vi "Get Temp Power Stage.vi"(8 "error in":errorcluster, 10 "?":T1, 11 "HSU MCU V2 Monitor CFG in":refnum<class "HSU MCU V2 CFG.lvclass">) -> (0 "error out":errorcluster, 2 "Temperature":dbl format="%#_g °C", 3 "HSU MCU V2 Monitor CFG out":refnum<class "HSU MCU V2 CFG.lvclass">)   [LabVIEW 2024, in "HSU MCU V2 CFG.lvclass"]
doc: "PCB temperature of MCUs power stage/MOSFETS"
uses:
  HSU MCU V2 CFG.lvclass
  MCU Selector.ctl
  HSU MCU V2 CFG.lvclass/HSU MCU V2 CFG.ctl
  Protocols/ICAN/ICAN.lvclass
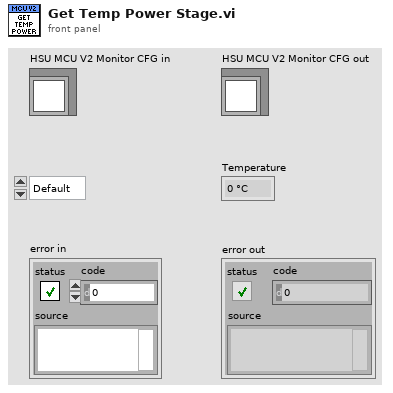
[diagram p1: front panel]
types:
  T1 = typedef "MCU Selector.ctl" = enum16{"Default", "MCU1", "MCU2", "MCU3", "MCU4", "MCU5", "MCU6", "MCU7", "MCU8", "ALL"}
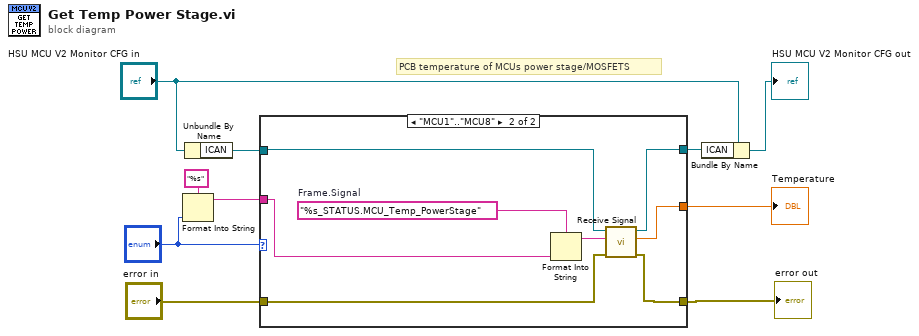
[diagram p0: block diagram]
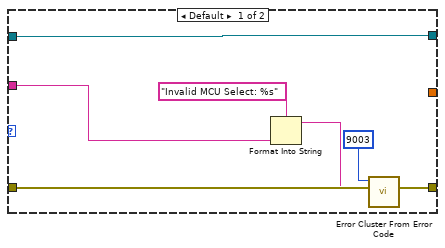
[diagram p2: hidden frame]
diagram:
  # "PCB temperature of MCUs power stage/MOSFETS"
  n1 = Format Into String(format string="%s", "?") -> (resulting string=w9:string)  [unwired: 2 in, 1 out]
  n2 = Unbundle By Name("HSU MCU V2 Monitor CFG in") -> ("ICAN"=w8:refnum<class "ICAN.lvclass">)
  n3 = case shown="\"MCU1\"..\"MCU8\"" "?" {
    tunnel: "error in" -> [w17 w23]
    tunnel: [w16 w22] -> w5
    tunnel: w9 -> [w12 w25]
    tunnel: w8 -> [w11 w24]
    tunnel: [w11 w21] -> w7
    tunnel: [_ w18] -> w6
    frame Default {
      n4 = Format Into String(format string="Invalid MCU Select: %s" ("error message (\"\")"), w12) -> (resulting string=w14:string)  [unwired: 2 in, 1 out]
      n5 = call <vilib>:"Error Cluster From Error Code.vi"("error in (no error)"=w17, "error message (\"\")"=w14, "error code (0)"=9003) -> ("error out"=w16:errorcluster)  [unwired: 6 in]
    }
    frame "MCU1".."MCU8" {
      w20 = "%s_STATUS.MCU_Temp_PowerStage"  # Frame.Signal
      n6 = Format Into String(format string=w20, w25) -> (resulting string=w19:string)  [unwired: 2 in, 1 out]
      n7 = call-dynamic "Receive Signal.vi"("error in"=w23, "Frame.Signal"=w19, "ICommunicate in"=w24) -> ("error out"=w22:errorcluster, "Value"=w18:dbl, "ICommunicate out"=w21:refnum<class "ICAN.lvclass">)  [unwired: 6 in]
    }
  }
  "Temperature" <- w6
  "error out" <- w5
  n8 = Bundle By Name(cluster="HSU MCU V2 Monitor CFG in", "ICAN"=w7) -> (→"HSU MCU V2 Monitor CFG out":refnum<class "HSU MCU V2 CFG.lvclass">)
